vi "Listener - Sobot.vi"() -> ()   [LabVIEW 2017]
uses:
  sobot structures/Z_Command.ctl
  sobot structures/XY_Commands.ctl
  sobot structures/General_Command.ctl
  sobot structures/ReturnDataStatus.ctl
  80253a44-10f1-4477-ae54-e8079e11bad8.vi
  35365326-f22b-4db8-b6bc-c4cae7e3b4d2.vi
  1f1e2b7e-f6f5-49aa-af42-c482bdb01d9c.vi
panel:
  out "String":string
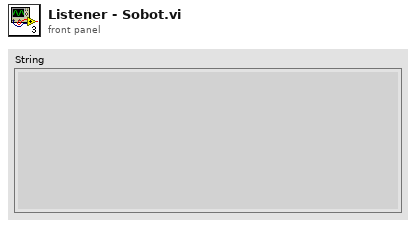
[diagram p1: front panel]
types:
  T1 = typedef "SoBot_CommandTypes.ctl" = enum16{"General_Command", "XY_Command", "Z_Command", "Plattform_Command"}
  T2 = typedef "General_Command.ctl" = enum16{"General_Stop", "General_StartSobotAutomatic", "General_StopSobotAutomatic", "General_TransferPoint", "General_Initialize", "General_SimpleMessage", "General_Ping"}
  T3 = typedef "ReturnDataStatus.ctl" = enum16{"AllOk", "Error"}
  T4 = typedef "XY_Commands.ctl" = enum16{"XY_Initialize", "XY_MoveToPosition", "XY_MarkTarget", "XY_LockMotors", "XY_UnlockMotors"}
  T5 = typedef "Z_Command.ctl" = enum16{"Z_Initialize", "Z_MoveToPosition", "Z_Focus", "Z_ReflectorPosition"}
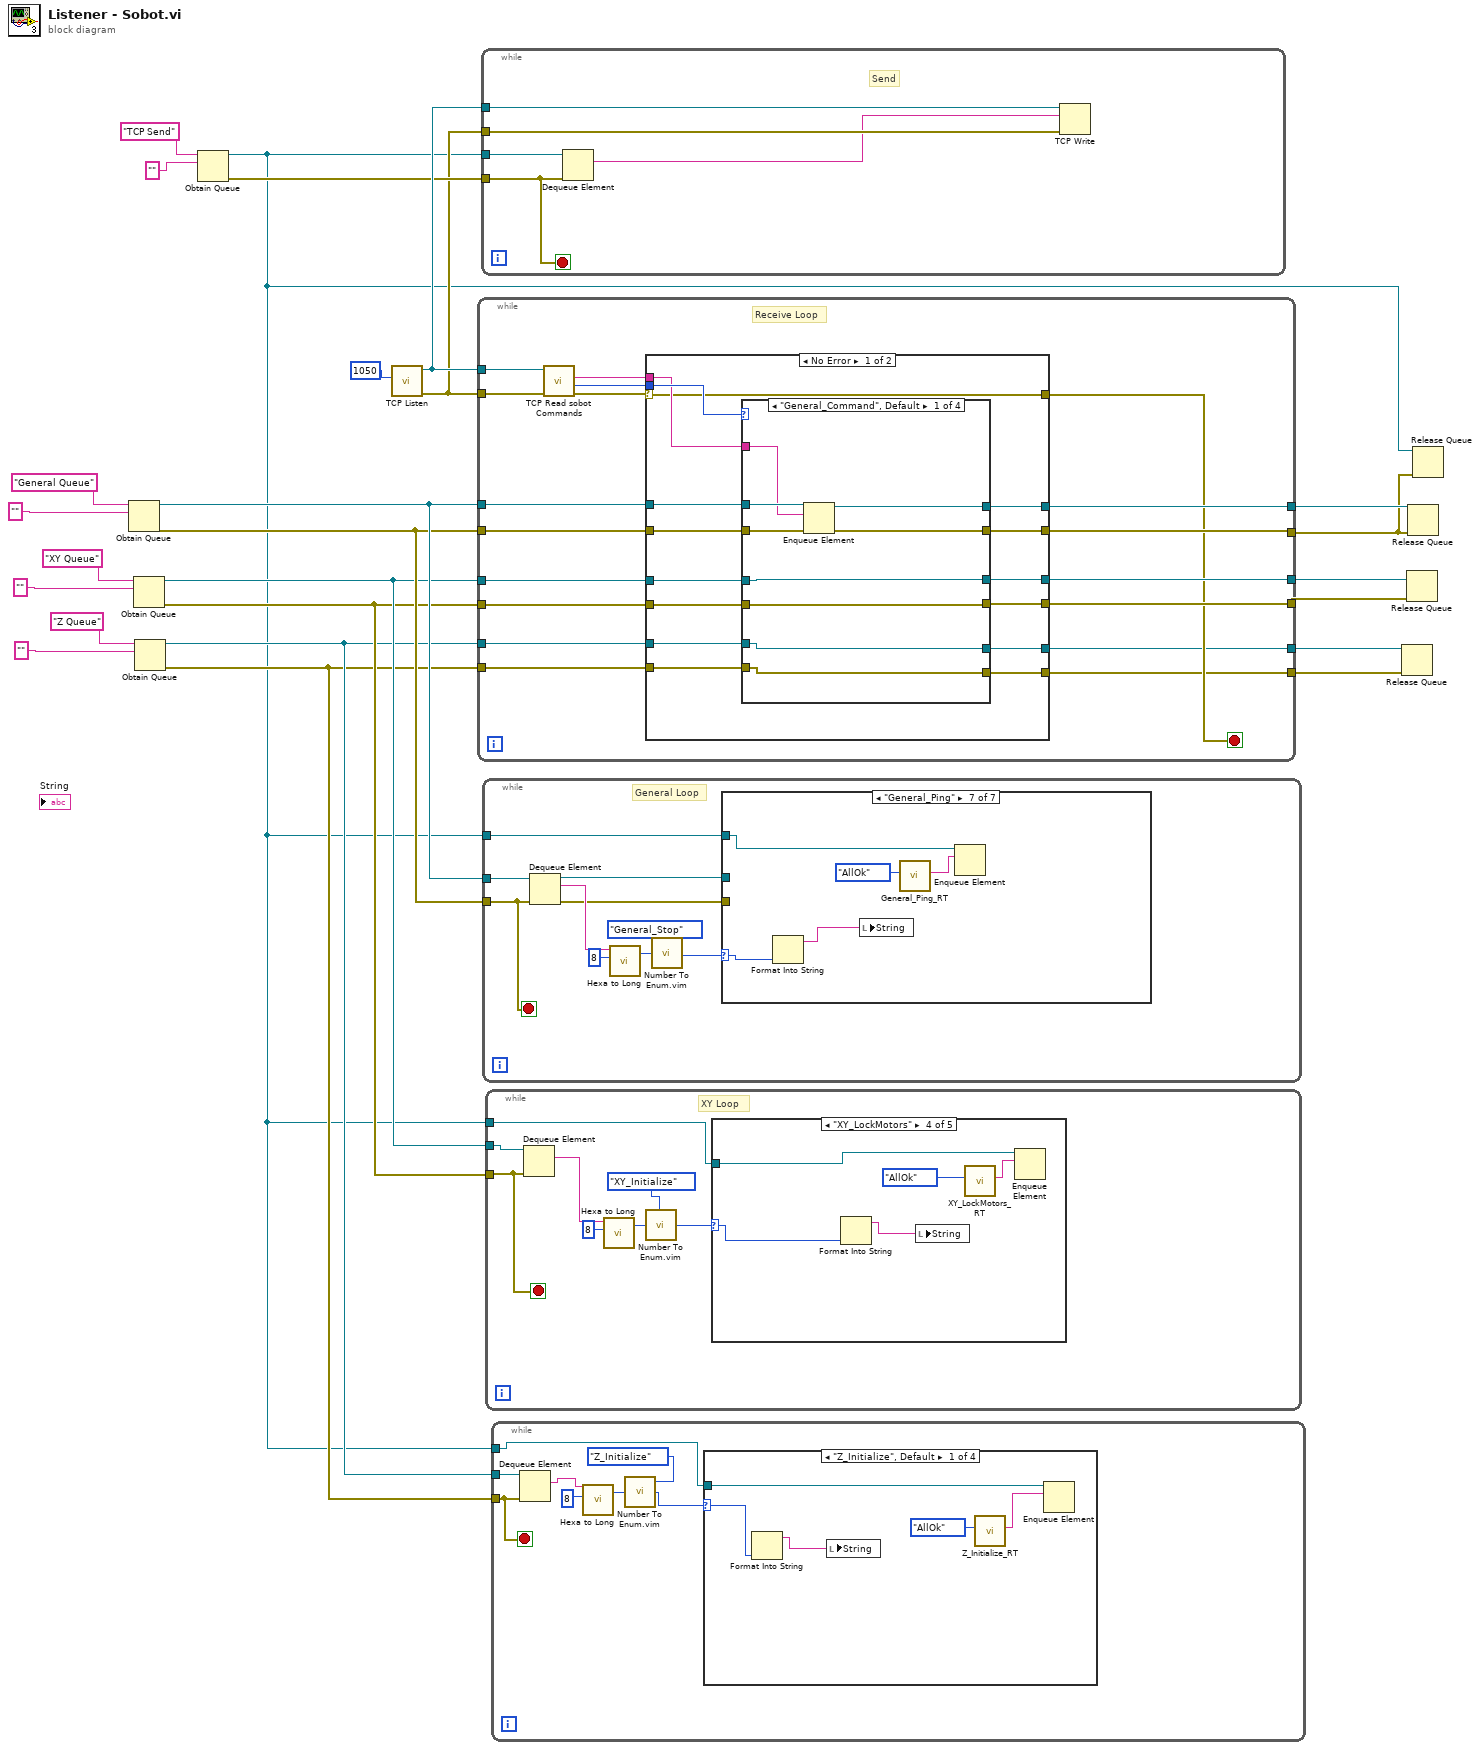
[diagram p0: block diagram]
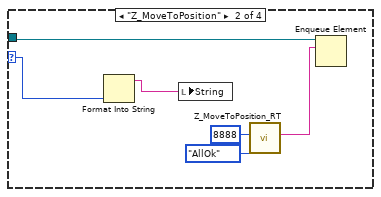
[diagram p2: hidden frame]
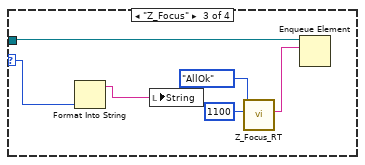
[diagram p3: hidden frame]
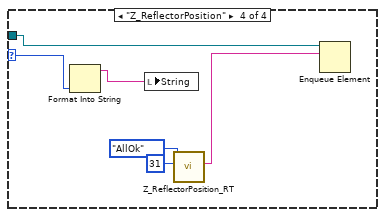
[diagram p4: hidden frame]
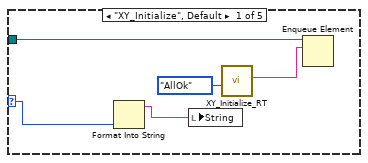
[diagram p5: hidden frame]
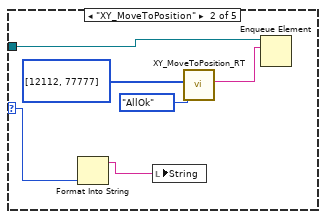
[diagram p6: hidden frame]
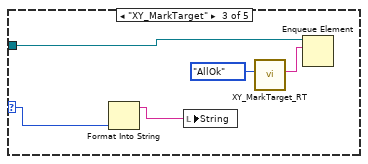
[diagram p7: hidden frame]
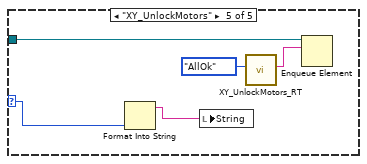
[diagram p8: hidden frame]
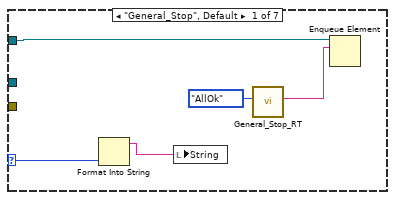
[diagram p9: hidden frame]
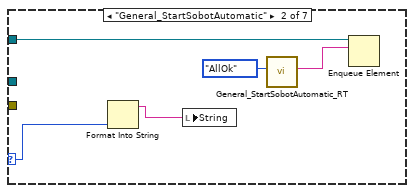
[diagram p10: hidden frame]
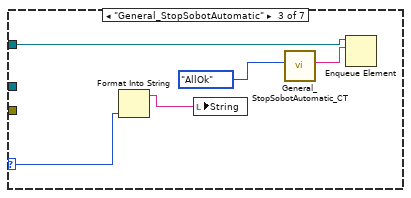
[diagram p11: hidden frame]
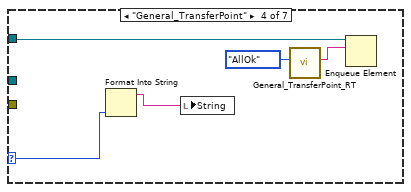
[diagram p12: hidden frame]
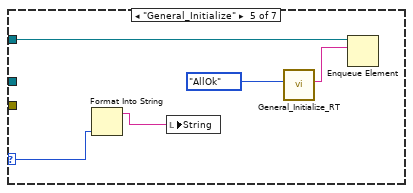
[diagram p13: hidden frame]
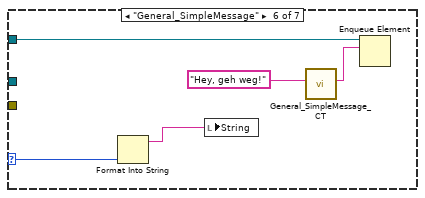
[diagram p14: hidden frame]
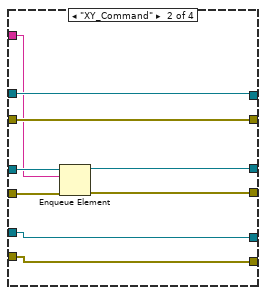
[diagram p15: hidden frame]
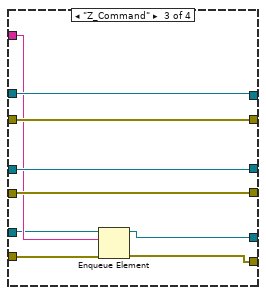
[diagram p16: hidden frame]
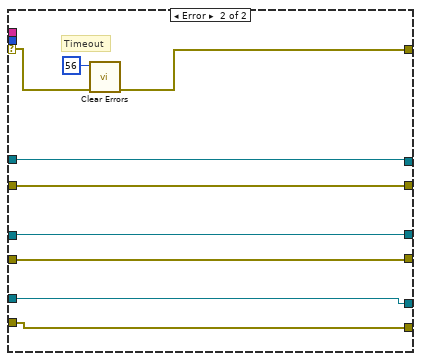
[diagram p18: hidden frame]
diagram:
  n1 = Obtain Queue(name (unnamed)="General Queue", element data type="" ("data out")) -> (queue out=w23:refnum<queue>, error out=w22:errorcluster)  [unwired: 3 in, 1 out]
  n2 = Obtain Queue(name (unnamed)="XY Queue", element data type="" ("data out")) -> (queue out=w15:refnum<queue>, error out=w14:errorcluster)  [unwired: 3 in, 1 out]
  n3 = Obtain Queue(name (unnamed)="Z Queue", element data type="" ("data out")) -> (queue out=w9:refnum<queue>, error out=w8:errorcluster)  [unwired: 3 in, 1 out]
  n4 = Obtain Queue(name (unnamed)="TCP Send", element data type="" ("name (unnamed)")) -> (queue out=w2:refnum<queue>, error out=w5:errorcluster)  [unwired: 3 in, 1 out]
  n5 = call <vilib>:"TCP Listen.vi"("port"=u16 1050) -> ("error out"=w4:errorcluster, "connection ID"=w7:refnum<k5>)  [unwired: 6 in, 3 out]
  n6 = while {
    tunnel: w4 -> [w43]
    tunnel: w7 -> [w42]
    tunnel: w23 -> [w40]
    tunnel: w22 -> [w38]
    tunnel: w15 -> [w36]
    tunnel: w14 -> [w35]
    tunnel: [w34] -> w18
    tunnel: [w33] -> w17
    tunnel: [w32] -> w16
    tunnel: [w31] -> w1
    tunnel: w9 -> [w29]
    tunnel: w8 -> [w28]
    tunnel: [w27] -> w11
    tunnel: [w26] -> w10
    stop <- w30 stop-if-true
    # "Receive Loop"
    n7 = call "TCP Read sobot Commands.vi"("error in (no error)"=w43, "TCP Network Connection in"=w42) -> ("error out"=w37:errorcluster, "SoBot_CommandTypes"=w41:T1, "data out"=w39:string)  [unwired: 6 in, 1 out]
    n8 = case shown="No Error" w37 {
      selector: w37 -> [w54 w96]
      tunnel: w41 -> [w58 _]
      tunnel: w40 -> [w57 w98]
      tunnel: w39 -> [w56 _]
      tunnel: w38 -> [w55 w97]
      tunnel: [w54 w95] -> w30
      tunnel: w36 -> [w53 w100]
      tunnel: w35 -> [w52 w99]
      tunnel: [w51 w100] -> w34
      tunnel: [w50 w99] -> w33
      tunnel: [w49 w98] -> w32
      tunnel: [w48 w97] -> w31
      tunnel: w29 -> [w47 w93]
      tunnel: w28 -> [w46 w92]
      tunnel: [w45 w93] -> w27
      tunnel: [w44 w92] -> w26
      frame No Error {
        n9 = case shown="\"General_Command\", Default" w58 {
          tunnel: w57 -> [w67 w72 w83 w89]
          tunnel: w56 -> [w65 w70 w81 _]
          tunnel: w55 -> [w66 w71 w82 w88]
          tunnel: w53 -> [w64 w76 w85 w91]
          tunnel: w52 -> [w63 w75 w84 w90]
          tunnel: [w64 w74 w85 w91] -> w51
          tunnel: [w63 w73 w84 w90] -> w50
          tunnel: [w62 w72 w83 w89] -> w49
          tunnel: [w61 w71 w82 w88] -> w48
          tunnel: w47 -> [w60 w69 w80 w87]
          tunnel: w46 -> [w59 w68 w79 w86]
          tunnel: [w60 w69 w78 w87] -> w45
          tunnel: [w59 w68 w77 w86] -> w44
          frame "General_Command", Default {
            n10 = Enqueue Element(queue=w67, element=w65, error in (no error)=w66) -> (queue out=w62:refnum<queue>, error out=w61:errorcluster)  [unwired: 1 in, 1 out]
          }
          frame "XY_Command" {
            n11 = Enqueue Element(queue=w76, element=w70, error in (no error)=w75) -> (queue out=w74:refnum<queue>, error out=w73:errorcluster)  [unwired: 1 in, 1 out]
          }
          frame "Z_Command" {
            n12 = Enqueue Element(queue=w80, element=w81, error in (no error)=w79) -> (queue out=w78:refnum<queue>, error out=w77:errorcluster)  [unwired: 1 in, 1 out]
          }
          frame "Plattform_Command" {
          }
        }
      }
      frame Error {
        # "Timeout"
        n13 = call <vilib>:"Clear Errors.vi"("error in (no error)"=w96, "specific error code to clear (0: all)"=56) -> ("error out"=w95:errorcluster)  [unwired: 4 in, 1 out]
      }
    }
  }
  n14 = while {
    tunnel: w7 -> [w105]
    tunnel: w2 -> [w104]
    tunnel: w5 -> [w101]
    tunnel: w4 -> [w103]
    stop <- w101 stop-if-true
    # "Send"
    n15 = Dequeue Element(queue=w104, error in (no error)=w101) -> (element=w102:string)  [unwired: 1 in, 3 out]
    n16 = TCP Write(connection ID=w105, data in=w102, error in (no error)=w103) -> ()  [unwired: 1 in, 3 out]
  }
  n17 = while {
    tunnel: w23 -> [w115]
    tunnel: w22 -> [w107]
    tunnel: w2 -> [w106]
    stop <- w107 stop-if-true
    # "General Loop"
    n18 = Dequeue Element(queue=w115, error in (no error)=w107) -> (queue out=w108:refnum<queue>, element=w114:string, error out=w109:errorcluster)  [unwired: 1 in, 1 out]
    n19 = call "Hexa to Long.vi"("Hexa"=w114, "Index"=8) -> ("Long"=w112:u32)  [unwired: 4 in]
    n20 = call "Number To Enum.vim"("number"=w112, "enum type"=General_Command."General_Stop" ("General_Command")) -> ("number as enum"=w110:T2)
    n21 = case shown="\"General_Ping\"" w110 {
      selector: w110 -> [w119 w124 w129 w134 w139 w144 w149]
      tunnel: w109 -> [_ _ _ _ _ _ _]
      tunnel: w108 -> [_ _ _ _ _ _ _]
      tunnel: w106 -> [w118 w122 w128 w133 w137 w143 w148]
      frame "General_Stop", Default {
        n22 = Format Into String(w119) -> (resulting string=w120:string)  [unwired: 3 in, 1 out]
        n23 = local write "String"(w120) -> ()
        n24 = call "General_Stop_RT.vi"("ReturnDataStatus"=ReturnDataStatus."AllOk") -> ("Command"=w117:string)  [unwired: 10 in]
        n25 = Enqueue Element(queue=w118, element=w117) -> ()  [unwired: 2 in, 3 out]
      }
      frame "General_StartSobotAutomatic" {
        n26 = Format Into String(w124) -> (resulting string=w125:string)  [unwired: 3 in, 1 out]
        n27 = local write "String"(w125) -> ()
        n28 = call "General_StartSobotAutomatic_RT.vi"("ReturnDataStatus"=ReturnDataStatus."AllOk") -> ("Command"=w121:string)  [unwired: 10 in]
        n29 = Enqueue Element(queue=w122, element=w121) -> ()  [unwired: 2 in, 3 out]
      }
      frame "General_StopSobotAutomatic" {
        n30 = Format Into String(w129) -> (resulting string=w130:string)  [unwired: 3 in, 1 out]
        n31 = local write "String"(w130) -> ()
        n32 = call "General_StopSobotAutomatic_CT.vi"("ReturnDataStatus"=ReturnDataStatus."AllOk") -> ("Command"=w127:string)  [unwired: 10 in]
        n33 = Enqueue Element(queue=w128, element=w127) -> ()  [unwired: 2 in, 3 out]
      }
      frame "General_TransferPoint" {
        n34 = Format Into String(w134) -> (resulting string=w135:string)  [unwired: 3 in, 1 out]
        n35 = local write "String"(w135) -> ()
        n36 = call "General_TransferPoint_RT.vi"("ReturnDataStatus"=ReturnDataStatus."AllOk") -> ("Command"=w132:string)  [unwired: 10 in]
        n37 = Enqueue Element(queue=w133, element=w132) -> ()  [unwired: 2 in, 3 out]
      }
      frame "General_Initialize" {
        n38 = Format Into String(w139) -> (resulting string=w140:string)  [unwired: 3 in, 1 out]
        n39 = local write "String"(w140) -> ()
        n40 = call "General_Initialize_RT.vi"("ReturnDataStatus"=ReturnDataStatus."AllOk") -> ("Command"=w136:string)  [unwired: 10 in]
        n41 = Enqueue Element(queue=w137, element=w136) -> ()  [unwired: 2 in, 3 out]
      }
      frame "General_SimpleMessage" {
        n42 = Format Into String(w144) -> (resulting string=w145:string)  [unwired: 3 in, 1 out]
        n43 = local write "String"(w145) -> ()
        n44 = call "General_SimpleMessage_CT.vi"("Message"="Hey, geh weg!") -> ("Command"=w142:string)  [unwired: 10 in]
        n45 = Enqueue Element(queue=w143, element=w142) -> ()  [unwired: 2 in, 3 out]
      }
      frame "General_Ping" {
        n46 = Format Into String(w149) -> (resulting string=w150:string)  [unwired: 3 in, 1 out]
        n47 = local write "String"(w150) -> ()
        n48 = call "General_Ping_RT.vi"("ReturnDataStatus"=ReturnDataStatus."AllOk") -> ("Command"=w147:string)  [unwired: 10 in]
        n49 = Enqueue Element(queue=w148, element=w147) -> ()  [unwired: 2 in, 3 out]
      }
    }
  }
  n50 = while {
    tunnel: w15 -> [w155]
    tunnel: w14 -> [w152]
    tunnel: w2 -> [w151]
    stop <- w152 stop-if-true
    # "XY Loop"
    n51 = Dequeue Element(queue=w155, error in (no error)=w152) -> (element=w158:string)  [unwired: 1 in, 3 out]
    n52 = call "Hexa to Long.vi"("Hexa"=w158, "Index"=8) -> ("Long"=w156:u32)  [unwired: 4 in]
    n53 = call "Number To Enum.vim"("number"=w156, "enum type"=XY_Commands."XY_Initialize" ("XY_Command")) -> ("number as enum"=w153:T4)
    n54 = case shown="\"XY_LockMotors\"" w153 {
      selector: w153 -> [w162 w168 w173 w178 w183]
      tunnel: w151 -> [w160 w164 w171 w177 w182]
      frame "XY_Initialize", Default {
        n55 = Format Into String(w162) -> (resulting string=w163:string)  [unwired: 3 in, 1 out]
        n56 = local write "String"(w163) -> ()
        n57 = call "XY_Initialize_RT.vi"("ReturnDataStatus"=ReturnDataStatus."AllOk") -> ("Command"=w159:string)  [unwired: 10 in]
        n58 = Enqueue Element(queue=w160, element=w159) -> ()  [unwired: 2 in, 3 out]
      }
      frame "XY_MoveToPosition" {
        n59 = Format Into String(w168) -> (resulting string=w169:string)  [unwired: 3 in, 1 out]
        n60 = local write "String"(w169) -> ()
        n61 = call "XY_MoveToPosition_RT.vi"("ReturnDataStatus"=ReturnDataStatus."AllOk", "Positon (X / Y)"=i32[] [12112, 77777]) -> ("Command"=w165:string)  [unwired: 9 in]
        n62 = Enqueue Element(queue=w164, element=w165) -> ()  [unwired: 2 in, 3 out]
      }
      frame "XY_MarkTarget" {
        n63 = Format Into String(w173) -> (resulting string=w174:string)  [unwired: 3 in, 1 out]
        n64 = local write "String"(w174) -> ()
        n65 = call "XY_MarkTarget_RT.vi"("ReturnDataStatus"=ReturnDataStatus."AllOk") -> ("Command"=w172:string)  [unwired: 10 in]
        n66 = Enqueue Element(queue=w171, element=w172) -> ()  [unwired: 2 in, 3 out]
      }
      frame "XY_LockMotors" {
        n67 = Format Into String(w178) -> (resulting string=w179:string)  [unwired: 3 in, 1 out]
        n68 = local write "String"(w179) -> ()
        n69 = call "XY_LockMotors_RT.vi"("ReturnDataStatus"=ReturnDataStatus."AllOk") -> ("Command"=w176:string)  [unwired: 10 in]
        n70 = Enqueue Element(queue=w177, element=w176) -> ()  [unwired: 2 in, 3 out]
      }
      frame "XY_UnlockMotors" {
        n71 = Format Into String(w183) -> (resulting string=w184:string)  [unwired: 3 in, 1 out]
        n72 = local write "String"(w184) -> ()
        n73 = call "XY_UnlockMotors_RT.vi"("ReturnDataStatus"=ReturnDataStatus."AllOk") -> ("Command"=w181:string)  [unwired: 10 in]
        n74 = Enqueue Element(queue=w182, element=w181) -> ()  [unwired: 2 in, 3 out]
      }
    }
  }
  n75 = while {
    tunnel: w9 -> [w192]
    tunnel: w8 -> [w186]
    tunnel: w2 -> [w185]
    stop <- w186 stop-if-true
    n76 = Dequeue Element(queue=w192, error in (no error)=w186) -> (element=w189:string)  [unwired: 1 in, 3 out]
    n77 = call "Hexa to Long.vi"("Hexa"=w189, "Index"=8) -> ("Long"=w190:u32)  [unwired: 4 in]
    n78 = call "Number To Enum.vim"("number"=w190, "enum type"=Z_Command."Z_Initialize" ("Z_Command")) -> ("number as enum"=w187:T5)
    n79 = case shown="\"Z_Initialize\", Default" w187 {
      selector: w187 -> [w196 w202 w208 w214]
      tunnel: w185 -> [w194 w201 w207 w213]
      frame "Z_Initialize", Default {
        n80 = Format Into String(w196) -> (resulting string=w197:string)  [unwired: 3 in, 1 out]
        n81 = local write "String"(w197) -> ()
        n82 = call "Z_Initialize_RT.vi"("ReturnDataStatus"=ReturnDataStatus."AllOk") -> ("Command"=w193:string)  [unwired: 10 in]
        n83 = Enqueue Element(queue=w194, element=w193) -> ()  [unwired: 2 in, 3 out]
      }
      frame "Z_MoveToPosition" {
        n84 = Format Into String(w202) -> (resulting string=w203:string)  [unwired: 3 in, 1 out]
        n85 = local write "String"(w203) -> ()
        n86 = call "Z_MoveToPosition_RT.vi"("ReturnDataStatus"=ReturnDataStatus."AllOk", "Z_Position"=8888) -> ("Command"=w200:string)  [unwired: 9 in]
        n87 = Enqueue Element(queue=w201, element=w200) -> ()  [unwired: 2 in, 3 out]
      }
      frame "Z_Focus" {
        n88 = Format Into String(w208) -> (resulting string=w209:string)  [unwired: 3 in, 1 out]
        n89 = local write "String"(w209) -> ()
        n90 = call "Z_Focus_RT.vi"("ReturnDataStatus"=ReturnDataStatus."AllOk", "Hight [mm]"=1100) -> ("Command"=w204:string)  [unwired: 9 in]
        n91 = Enqueue Element(queue=w207, element=w204) -> ()  [unwired: 2 in, 3 out]
      }
      frame "Z_ReflectorPosition" {
        n92 = Format Into String(w214) -> (resulting string=w215:string)  [unwired: 3 in, 1 out]
        n93 = local write "String"(w215) -> ()
        n94 = call "Z_ReflectorPosition_RT.vi"("ReturnDataStatus"=ReturnDataStatus."AllOk", "ReflectorPosition"=31) -> ("Command"=w212:string)  [unwired: 9 in]
        n95 = Enqueue Element(queue=w213, element=w212) -> ()  [unwired: 2 in, 3 out]
      }
    }
  }
  n96 = Release Queue(queue=w11, error in (no error)=w10) -> ()  [unwired: 1 in, 3 out]
  n97 = Release Queue(queue=w18, error in (no error)=w17) -> ()  [unwired: 1 in, 3 out]
  n98 = Release Queue(queue=w16, error in (no error)=w1) -> ()  [unwired: 1 in, 3 out]
  n99 = Release Queue(queue=w2, error in (no error)=w1) -> ()  [unwired: 1 in, 3 out]
